vi "Plink.vi"(7 "Console":refnum<vi>, 8 "error in":errorcluster, 9 "Command(s) to Execute":string="pwd", 10 "Host":string="172.22.11.2", 11 "plink path":path=path "bin/plink.exe") -> (0 "error out":errorcluster, 1 "return code":i32, 2 "Errors":string, 3 "Command Return Value(s)":string, 5 "Command Executed":string)   [LabVIEW 2016]
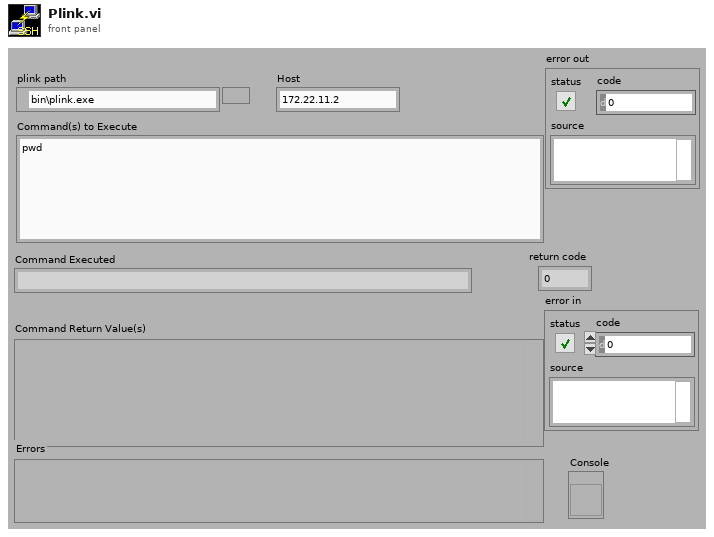
[diagram p1: front panel]
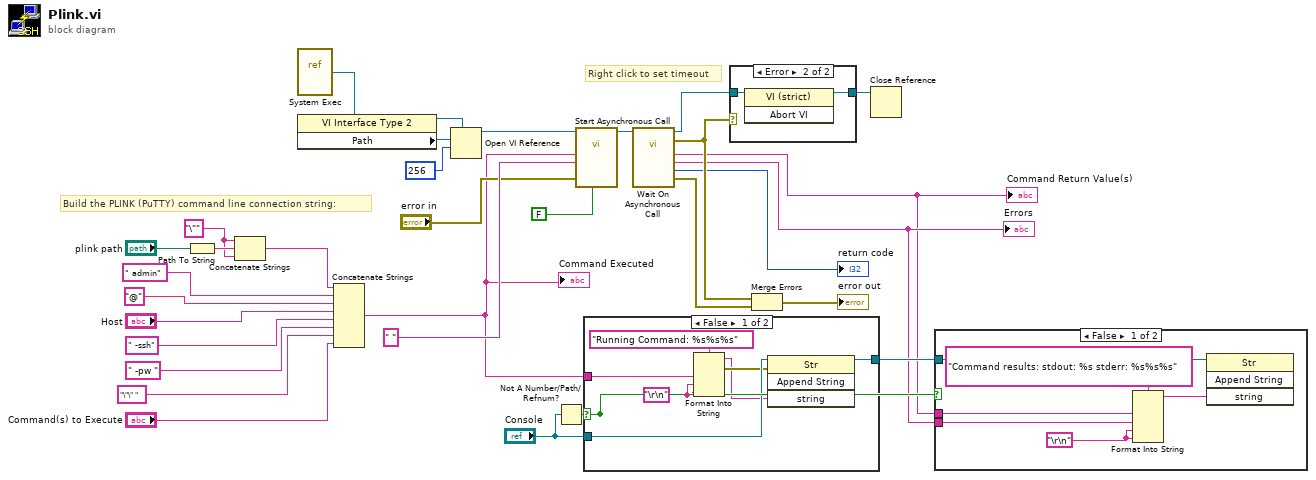
[diagram p0: block diagram]
diagram:
  w23 = "\"" ("string")
  # "Right click to set timeout"
  # "Build the PLINK (PuTTY) command line connection string:"
  n1 = Path To String(path="plink path") -> (string=w24:string)
  n2 = Concatenate Strings(w23, w24, w23) -> (w22:string)
  n3 = vi-ref <vilib>:"System Exec.vi"() -> (w20:refnum<vi>)
  n4 = property class="VI Interface Type 2"(reference=w20) -> (reference out=w17:refnum<vi>, "Path"=w19:path)  [unwired: 1 in, 1 out]
  n5 = Concatenate Strings(w22, " admin" ("Username"), "@" ("string"), "Host", " -ssh", " -pw " ("string"), "\"\" " ("Password"), "Command(s) to Execute") -> (w6:string)
  "Command Executed" <- w6
  n6 = Open VI Reference(type specifier VI Refnum (for type only)=w17, vi path=w19, options=256) -> (vi reference=w21:refnum<vi>)  [unwired: 3 in, 1 out]
  n7 = Not A Number/Path/Refnum?(number/path/refnum="Console") -> (NaN/Path/Refnum?=w4:bool)
  n8 = call-by-ref "Start Asynchronous Call"(reference=w21, "run minimized? (F)"=FALSE ("Hide DOS\nWindow?"), "error in (no error)"="error in", "standard input"=" ", "command line"=w6) -> (reference out=w16:refnum<vi>)  [unwired: 5 in, 5 out]
  n9 = case shown="False" w4 {
    tunnel: "Console" -> [w39 _]
    tunnel: w6 -> [w37 _]
    tunnel: [w34 _] -> w3
    frame False {
      w33 = "\r\n"
      n10 = Format Into String(format string="Running Command: %s%s%s" ("string"), w37, w33, w33) -> (resulting string=w35:string, error out=w36:errorcluster)  [unwired: 2 in]
      n11 = invoke class="Str" method="Append String"(reference=w39, error in=w36, "string"=w35) -> (reference out=w34:refnum<vi>)  [unwired: 1 in, 3 out]
    }
    frame True {
    }
  }
  n12 = call-by-ref "Wait On Asynchronous Call"(reference=w16) -> (reference out=w11:refnum<vi>, error out=w10:errorcluster, 0:"error out"=w13:errorcluster, "return code"=→"return code":i32, "standard error"=w2:string, "standard output"=w1:string)  [unwired: 9 in]
  "Command Return Value(s)" <- w1
  "Errors" <- w2
  n13 = case shown="Error" w10 {
    tunnel: [w40 w42] -> w12
    tunnel: w11 -> [w40 w41]
    frame No Error {
    }
    frame Error {
      n14 = invoke class="VI (strict)" method="Abort VI"(reference=w41) -> (reference out=w42:refnum<vi>)  [unwired: 2 in, 2 out]
    }
  }
  n15 = Merge Errors(w10, w13) -> (→"error out":errorcluster)
  n16 = Close Reference(reference=w12) -> ()  [unwired: 1 in, 1 out]
  n17 = case shown="False" w4 {
    tunnel: w3 -> [w46 _]
    tunnel: w2 -> [w45 _]
    tunnel: w1 -> [w44 _]
    frame False {
      w43 = "\r\n"
      n18 = Format Into String(format string="Command results: stdout: %s stderr: %s%s%s" ("string"), w44, w45, w43, w43) -> (resulting string=w47:string)  [unwired: 2 in, 1 out]
      n19 = invoke class="Str" method="Append String"(reference=w46, "string"=w47) -> ()  [unwired: 2 in, 4 out]
    }
    frame True {
    }
  }
